vi "Projection Mode Read.vi"(8 "error in (no error)":errorcluster, 11 "3D Plot.lvclass in":refnum<class "3D Plot.lvclass">) -> (0 "error out":errorcluster, 1 "Projection Mode":enum16{"Orthographic", "Perspective"}(ring), 3 "3D Plot.lvclass out":refnum<class "3D Plot.lvclass">)   [LabVIEW 2020, in "3D Plot.lvclass"]
uses:
  <vilib>/Math Plots/3D Math Plots/3D Plot/3D Plot/3D Plot.lvclass
  <vilib>/Math Plots/3D Math Plots/3D Plot/3D Plot/3D Plot.lvclass/3D Plot.ctl
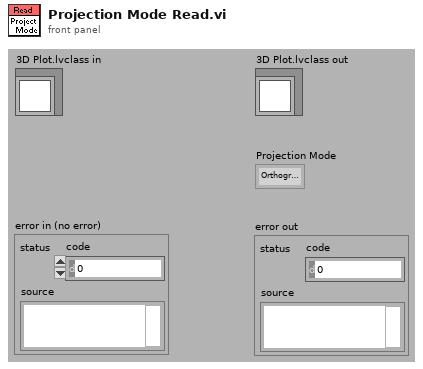
[diagram p1: front panel]
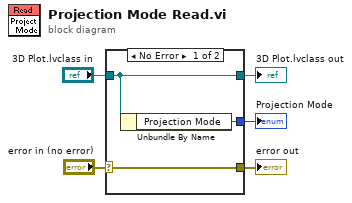
[diagram p0: block diagram]
diagram:
  n1 = case shown="No Error" "error in (no error)" {
    selector: "error in (no error)" -> [w6 w9]
    tunnel: [w8 _] -> w5
    tunnel: "3D Plot.lvclass in" -> [w7 w10]
    tunnel: [w7 w10] -> w3
    tunnel: [w6 w9] -> w1
    frame No Error {
      n2 = Unbundle By Name(w7) -> ("Projection Mode"=w8:enum16{"Orthographic", "Perspective"})
    }
    frame Error {
    }
  }
  "Projection Mode" <- w5
  "error out" <- w1
  "3D Plot.lvclass out" <- w3
